vi "Get Actuator AO DAQmx Ref.vi"(8 "error in (no error)":errorcluster, 10 "AO IOName Idx":i32, 11 "DAQ in":refnum<class "DAQ.lvclass">) -> (0 "error out":errorcluster, 2 "AO Actuator DAQmx Task":refnum<k21>, 3 "DAQ out":refnum<class "DAQ.lvclass">)   [LabVIEW 2017, in "DAQ.lvclass"]
doc: "Developed by Kevin Thompson\nkevin@thompsonengineering.net\n\nCopyright 2018-2020\nThompson Engineering, LLC"
uses:
  DAQ.lvclass
  DataTypes/TD AO Channel--cluster.ctl
  DataTypes/TD DataValueConversion--cluster.ctl
  DAQ.lvclass/DAQ.ctl
  Accessors/Get DAQNodes Dict.vi
  Accessors/Get DAQ Settings.vi
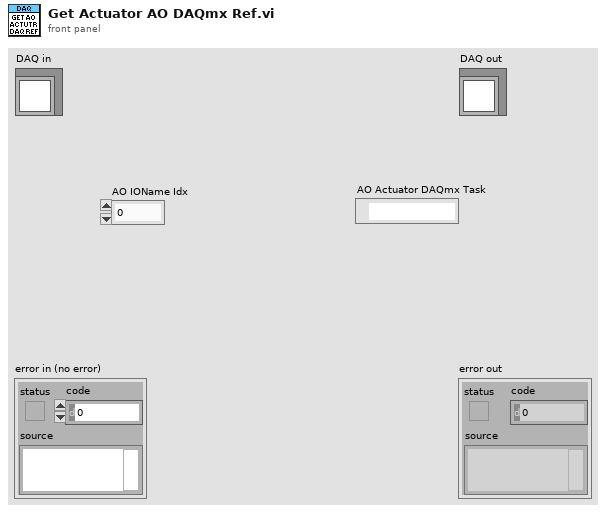
[diagram p1: front panel]
types:
  T1 = typedef "DAQ.lvclass/TD AO Channel--cluster.ctl" = cluster{"DevName":string, "IOName":string, "IOPath":string, "SchemName":string, "Vmin":dbl, "Vmax":dbl, "Conversion":T2, "DAQmx Task":refnum<k21>}
  T2 = typedef "DAQ.lvclass/TD DataValueConversion--cluster.ctl" = cluster{"MaxSignal":dbl, "MinSignal":dbl, "MaxEngUnit":dbl, "MinEngUnit":dbl, "ScaleOffset":dbl, "negate":bool}
  T3 = typedef "TD Dynamic CVT DVR--ref.ctl" = refnum<data-value>
  T4 = typedef "DAQ.lvclass/TD DAQ Settings--cluster.ctl" = cluster{"Simulate DAQ":bool, "DI Settings":T5[], "AI Settings":T6[], "Relay IONames":string[], "AO IONames":string[], "AO NChan SingleTask":bool}
  T5 = typedef "DAQ.lvclass/TD DI Instrument Settings--cluster.ctl" = cluster{"Disable":bool, "DI TaskName":string, "DI RefreshIntv":i32}
  T6 = typedef "DAQ.lvclass/TD AI Instrument Settings--cluster.ctl" = cluster{"Disable":bool, "AI TaskName":string, "AI InstSettings":T7, "SimAI Ranges":T8}
  T7 = typedef "DAQ.lvclass/TD AI InstSettings--cluster.ctl" = cluster{"DaqRate":dbl, "NumSamples":i32}
  T8 = typedef "DAQ.lvclass/TD SimAI Ranges--cluster.ctl" = cluster{"lo":dbl, "hi":dbl}
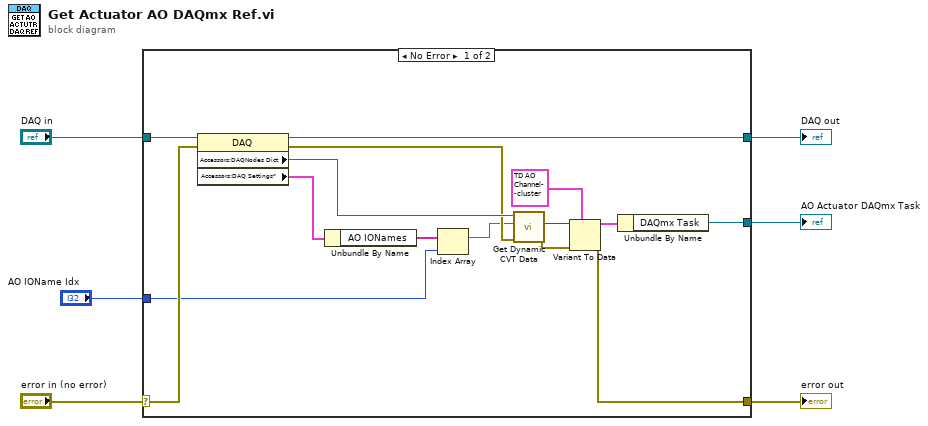
[diagram p0: block diagram]
diagram:
  n1 = case shown="No Error" "error in (no error)" {
    selector: "error in (no error)" -> [w10 w23]
    tunnel: [w16 w23] -> w5
    tunnel: [w20 w22] -> w3
    tunnel: "DAQ in" -> [w21 w22]
    tunnel: [w13 _] -> w2
    tunnel: "AO IOName Idx" -> [w7 _]
    frame No Error {
      n2 = property class="DAQ"(reference=w21, error in=w10) -> (reference out=w20:refnum<class "DAQ.lvclass">, error out=w9:errorcluster, "Accessors:DAQNodes Dict"=w19:T3, "Accessors:DAQ Settings*"=w12:T4)
      n3 = Unbundle By Name(w12) -> ("AO IONames"=w11:string[])
      n4 = Index Array(array=w11, index=w7) -> (element=w8:string)
      n5 = call <vilib>:"Get Dynamic CVT Data.vi"("error in (no error)"=w9, "DataName"=w8, "dCVT DVR"=w19) -> ("error out"=w17:errorcluster, "value"=w18:variant)  [unwired: 5 in, 2 out]
      n6 = Variant To Data(error in=w17, type=T1 {"DevName"="", "IOName"="", "IOPath"="", "SchemName"="", "Vmin"=0.0, "Vmax"=0.0, "Conversion"={"MaxSignal"=0.0, "MinSignal"=0.0, "MaxEngUnit"=0.0, "MinEngUnit"=0.0, "ScaleOffset"=0.0, "negate"=FALSE}, "DAQmx Task"=""} ("AO"), Variant=w18) -> (data=w14:T1, error out=w16:errorcluster)
      n7 = Unbundle By Name(w14) -> ("DAQmx Task"=w13:refnum<k21>)
    }
    frame Error {
    }
  }
  "error out" <- w5
  "DAQ out" <- w3
  "AO Actuator DAQmx Task" <- w2
